vi "ADS1015 Example.vi"() -> ()   [LabVIEW 2014]
uses:
  <vilib>/myRIO/Instrument Drivers/Onboard IO/DIO/typedefs/DIO Reference.ctl
  <vilib>/myRIO/Common/Instrument Driver Framework/Utilities/typedefs/myRIO Generic Hardware Reference.ctl
  <vilib>/myRIO/Common/Instrument Driver Framework/Utilities/typedefs/Hardware Version Enum.ctl
  <vilib>/myRIO/Common/Instrument Driver Framework/Utilities/typedefs/myRIO v1.0 Reference.ctl
  <vilib>/myRIO/Common/Instrument Driver Framework/Utilities/typedefs/Generic FPGA Reference.ctl
  <vilib>/myRIO/Common/Instrument Driver Framework/myRIO v1.0/DIO/typedefs/DIO Channels List.ctl
  <vilib>/myRIO/Common/Instrument Driver Framework/myRIO v1.0/DIO/typedefs/DIO Channels Enum.ctl
  <vilib>/userdefined/High Color/nirio_resource_hc.ctl
  <vilib>/myRIO/Common/Instrument Driver Framework/Utilities/vis/Is FPGA Ref Available.vi
  <vilib>/myRIO/Common/Instrument Driver Framework/myRIO v1.0/DIO/vis/myRIO v1.1 Open DIO.vi
  <vilib>/myRIO/Instrument Drivers/Onboard IO/DIO/vis/Write.vi
  <vilib>/myRIO/Common/Instrument Driver Framework/Utilities/vis/Validate Channels.vi
  <vilib>/myRIO/Common/Instrument Driver Framework/myRIO v1.0/DIO/vis/myRIO v1.0 Reserve DIO.vi
  <vilib>/MakerHub/LINX/Public/Utilities/Check Channel.vi
  <vilib>/myRIO/Common/Instrument Driver Framework/myRIO v1.0/Resource Manager/vis/myRIO v1.0 Reserve Channel List.vi
  <vilib>/myRIO/Common/Instrument Driver Framework/myRIO v1.0/DIO/vis/myRIO v1.0 Build MUX Configuration DIO.vi
  <vilib>/myRIO/Common/Instrument Driver Framework/myRIO v1.0/Resource Manager/vis/myRIO v1.0 Reserve Channel.vi
  <vilib>/myRIO/Common/Instrument Driver Framework/myRIO v1.0/Resource Manager/vis/myRIO v1.0 Unreserve Channel.vi
  <vilib>/myRIO/Common/Instrument Driver Framework/myRIO v1.0/Resource Manager/vis/myRIO v1.0 Create Configuration List.vi
  <vilib>/myRIO/Common/Instrument Driver Framework/myRIO v1.0/Resource Manager/vis/myRIO v1.0 Build Mutex Name.vi
  <vilib>/Utility/VariantDataType/GetNumericInfo.vi
  <vilib>/Utility/error.llb/Error Cluster From Error Code.vi
  <vilib>/myRIO/Common/Instrument Driver Framework/myRIO v1.0/myRIO v1.1 Open.vi
  <vilib>/myRIO/Common/Instrument Driver Framework/Utilities/vis/IO Manager.vi
  <vilib>/myRIO/Common/Instrument Driver Framework/Utilities/vis/Configuration Manager.vi
  <vilib>/myRIO/Common/Instrument Driver Framework/myRIO v1.0/Resource Manager/vis/myRIO v1.0 Configure IO.vi
  <vilib>/myRIO/Common/Instrument Driver Framework/myRIO v1.0/myRIO v1.0 Close.vi
  <vilib>/myRIO/Common/Instrument Driver Framework/myRIO v1.0/DIO/vis/myRIO v1.0 Write DIO.vi
  <vilib>/MakerHub/LINX/Public/Utilities/Open Local.vi
  <vilib>/MakerHub/LINX/Private/Utilties/Generate Error.vi
  <vilib>/MakerHub/LINX/Private/Local IO/LinxI2cOpen.vi
  <vilib>/myRIO/Express VI/Onboard IO/DO/DO Express VI.xnode
  <vilib>/myRIO/Instrument Drivers/Onboard IO/DIO/vis/myRIO DIO Open.xnode
  <vilib>/MakerHub/LINX/LMH-LINX.lvlib
  <vilib>/myRIO/Instrument Drivers/Onboard IO/DIO/DIO.lvlib
panel:
  out "Resolutions":dbl[](array[numeric]) format="%.3f V"
  out "Voltages":dbl[](array[numeric]) format="%.3f V"
  in  "I2C Slave Address":u8=72 format="%x"
  in  "I2C Channel":u8=1
  out "Error Out":errorcluster
  out "Device Name":string
  out "ToF Loop Rate":u32
  in  "Wait (ms)":u32=10
  in  "Stop":bool
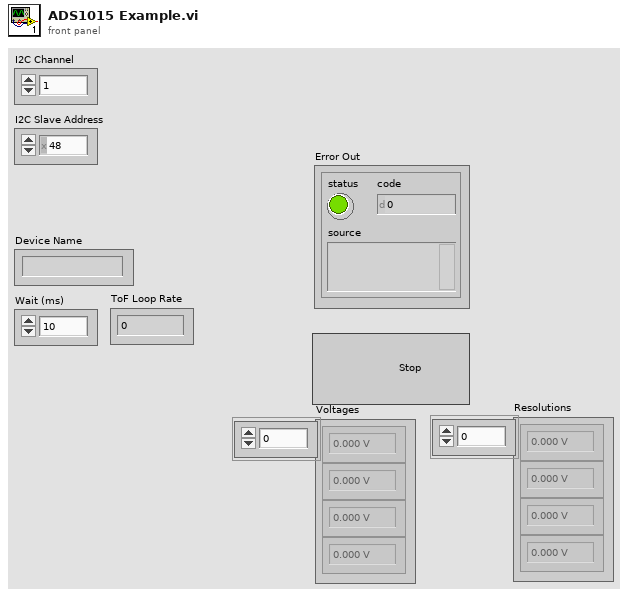
[diagram p1: front panel]
types:
  T1 = typedef "LMH-LINX.lvlib/LINX Ref.ctl" = cluster{"IO":T2, "Interface":T3, "LINX Device Config":T4}
  T2 = typedef "LMH-LINX.lvlib/Platform.ctl" = enum16{"Remote", "Local"}
  T3 = typedef "LMH-LINX.lvlib/Interface.ctl" = enum16{"Serial", "TCP"}
  T4 = typedef "LMH-LINX.lvlib/Device.lvlib/LINX Device Config.ctl" = cluster{"Interface":T3, "COM Port":refnum<visa-resource-name>, "TCP Configuration":T5, "Device Family":u8, "Device ID":u8, "Device Name":string, "TCP Ref":refnum<k5>, "Channels":T6}
  T5 = typedef "LMH-LINX.lvlib/Device.lvlib/TCP Config.ctl" = cluster{"IP Address":string, "Port":u16}
  T6 = typedef "LMH-LINX.lvlib/Channels.ctl" = cluster{"DI":u8[], "DO":u8[], "AI":u8[], "AO":u8[], "PWM":u8[], "QE":u8[], "UART":u8[], "I2C 2":u8[], "SPI":u8[], "CAN":u8[], "Servo":u8[], "AI Ref (V)":dbl, "AI Resolution (Bits)":u8, "AO Ref (V)":dbl, "AO Resolution (Bits)":u8}
  T7 = typedef "ADS1015 Config Options.ctl" = cluster{"I2C":cluster{"Slave Address":u8, "Channel":u8}, "ADC":cluster{"Channel":u8, "Expected Range (Programmable Gain Amplifier)":u8, "Sampling Mode":u8, "Sampling Rate":u8, "Comparator Mode":u8, "Comparator Polarity":u8, "Latching Comparator":u8, "Comparator Queue & Disable":u8}}
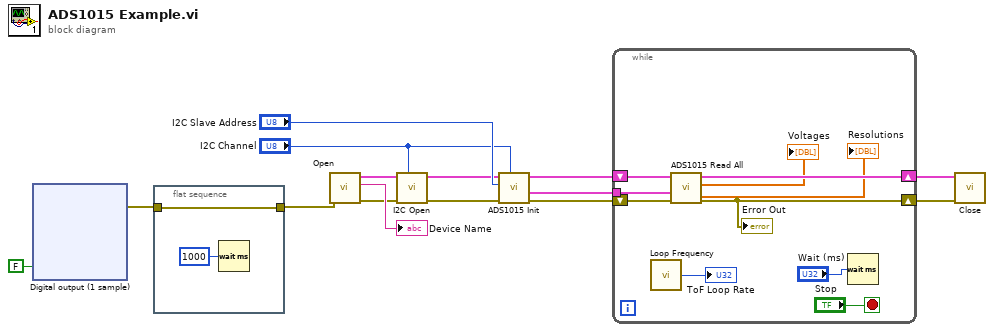
[diagram p0: block diagram]
diagram:
  n1 = xnode "Digital output (1 sample)"("Sensor Power (B/DIO7 (Pin 25))"=FALSE) -> ("error out"=w10:errorcluster)  [unwired: 1 in]
  n2 = flat-sequence {
    tunnel: w10 -> [w17]
    tunnel: [w17] -> w9
    frame #0 {
      n3 = Wait (ms)(milliseconds to wait=u32 1000) -> ()  [unwired: 1 out]
    }
  }
  n4 = call-poly <vilib>:"Open.vi"("Error In"=w9) -> ("Error Out"=w13:errorcluster, "Device Name"=→"Device Name":string, "LINX Resource"=w14:T1)  [unwired: 8 in]
  n5 = call <vilib>:"I2C Open.vi"("I2C Channel (0)"="I2C Channel", "Error In"=w13, "LINX Resource"=w14) -> ("Error Out"=w5:errorcluster, "LINX Resource"=w6:T1)  [unwired: 7 in]
  n6 = call "ADS1015 Init.vi"("I2C Channel"="I2C Channel", "error in (no error)"=w5, "I2C Slave Address"="I2C Slave Address", "LINX Resource in"=w6) -> ("error out"=w4:errorcluster, "ADS1015 Config Options"=w1:T7, "LINX Resource out"=w3:T1)  [unwired: 5 in]
  n7 = while {
    shift-right: [w22] -> w12
    shift-left: w3 -> [w25]
    shift-right: [w21] -> w11
    shift-left: w4 -> [w24]
    tunnel: w1 -> [w20]
    stop <- "Stop" stop-if-true
    n8 = call <vilib>:"Loop Frequency.vi"() -> ("Loop Rate (Hz)"=→"ToF Loop Rate":u32)
    n9 = call "ADS1015 Read All.vi"("error in (no error)"=w24, "ADS1015 Config Options"=w20, "LINX Resource in"=w25) -> ("error out"=w21:errorcluster, "Voltages"=→"Voltages":dbl[], "LINX Resource"=w22:T1, "Resolutions"=→"Resolutions":dbl[])  [unwired: 5 in]
    "Error Out" <- w21
    n10 = Wait (ms)(milliseconds to wait="Wait (ms)") -> ()  [unwired: 1 out]
  }
  n11 = call <vilib>:"Close.vi"("Error In"=w11, "LINX Resource"=w12) -> ()  [unwired: 9 in, 1 out]
